vi "DGML Container String from FQN.vi"(8 "error in (no error)":errorcluster, 11 "FQN Array":string[](array[string])) -> (0 "error out":errorcluster, 2 "Unowned?":bool, 3 "DGML Strings":string[](array[string]))   [LabVIEW 2018, in "Path and String Processing.lvlib"]
uses:
  Path and string processing/Path and String Processing.lvlib
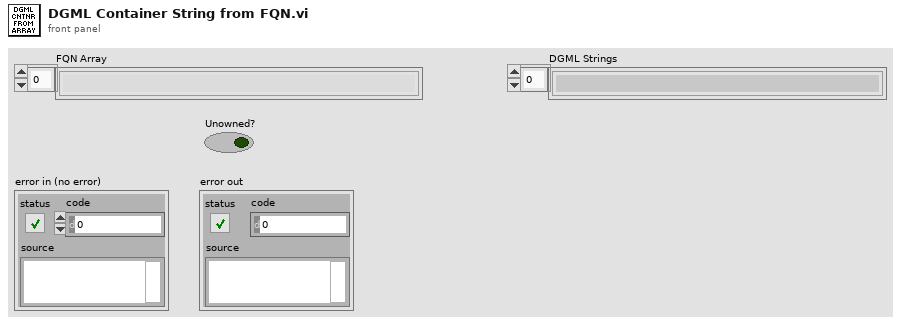
[diagram p1: front panel]
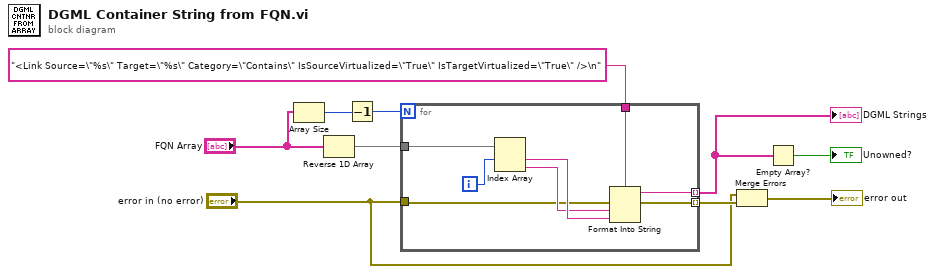
[diagram p0: block diagram]
diagram:
  n1 = Array Size(array="FQN Array") -> (size(s)=w5:i32)
  n2 = Reverse 1D Array(array="FQN Array") -> (reversed array=w4:string[])
  n3 = Decrement(x=w5) -> (x-1=w6:i32)
  n4 = for {
    N: w6 -> [_]
    tunnel: w4 -> [w16]
    tunnel: "<Link Source=\"%s\" Target=\"%s\" Category=\"Contains\" IsSourceVirtualized=\"True\" IsTargetVirtualized=\"True\" />\n" ("format string") -> [w18]
    tunnel: [w17] -> w7 mode=indexing
    tunnel: "error in (no error)" -> [w11]
    tunnel: [w12] -> w9 mode=indexing
    i -> [w15]
    n5 = Index Array(array=w16, index #1=w15) -> (element #1=w14:string, element #2=w13:string)  [unwired: 1 in]
    n6 = Format Into String(format string=w18, error in=w11, w13, w14) -> (resulting string=w17:string, error out=w12:errorcluster)  [unwired: 1 in]
  }
  "DGML Strings" <- w7
  n7 = Merge Errors("error in (no error)", w9) -> (→"error out":errorcluster)
  n8 = Empty Array?(array=w7) -> (empty?=→"Unowned?":bool)
